vi "Open WorkBook.vi"(2 "error in (no error)":errorcluster caption="错误输入（无错误）", 3 "Filename of Workbook":string caption="工作簿文件名", 4 "Excel._Application":refnum<k7>) -> (0 "error out":errorcluster caption="错误输出", 1 "Excel._Workbook":refnum<k7>)   [LabVIEW 2017]
doc: "按名称打开工作簿。将应用程序引用句柄作为输入。如尚未连接名称或者字符串长度为零，将打开一个新的工作簿，否则会将指定工作簿添加至工作簿对象集合。"
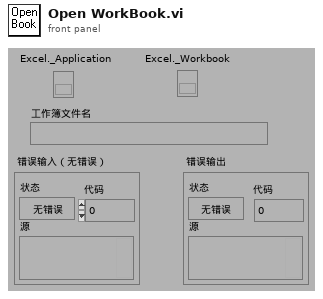
[diagram p1: front panel]
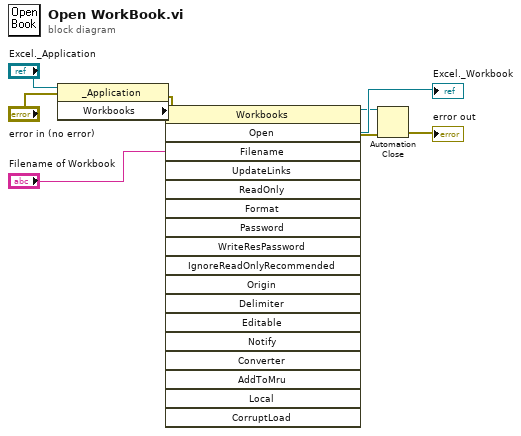
[diagram p0: block diagram]
diagram:
  n1 = property class="_Application"(reference="Excel._Application", error in="error in (no error)") -> (error out=w6:errorcluster, "Workbooks"=w7:refnum<k7>)  [unwired: 1 out]
  n2 = invoke class="Workbooks" method="Open"(reference=w7, error in=w6, "Filename"="Filename of Workbook") -> (reference out=w2:refnum<k7>, error out=w4:errorcluster, "Open"=→"Excel._Workbook":refnum<k7>)  [unwired: 15 in, 15 out]
  n3 = Automation Close(3:w4, 5:w2) -> (0:→"error out":errorcluster)
